vi "HTTPS Connection Callback.vi"(7 "Owner":refnum<class>, 8 "error in (no error)":errorcluster, 9 "Context":variant, 10 "Connection State":T1, 11 "Connection":refnum<class "Connection.lvclass">) -> (0 "error out":errorcluster)   [LabVIEW 2020, in "HTTP Server.lvlib" / "Server.lvclass"]
uses:
  Server.lvclass
  HTTP TCP Client/HTTP TCP Client.lvclass
  lv-stream/stream/Connection/Connection.lvclass
  lv-stream/stream/Connection State.ctl
  lv-stream/stream/Stream.lvlib
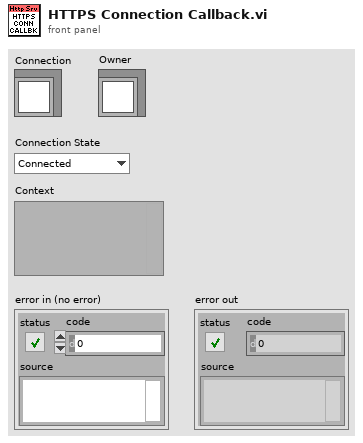
[diagram p1: front panel]
types:
  T1 = typedef "Stream.lvlib/Connection State.ctl" = enum16{"Connected", "Disconnected"}
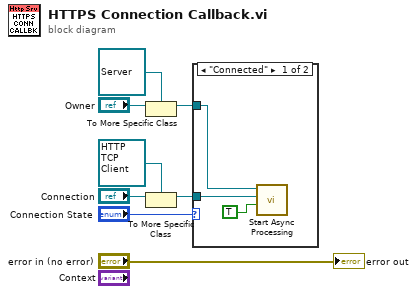
[diagram p0: block diagram]
diagram:
  n1 = To More Specific Class(target class=refnum<class "Server.lvclass"> refnum ("HTTP.lvlib:Server.lvclass"), reference="Owner") -> (specific class reference=w5:refnum<class "Server.lvclass">)  [unwired: 1 in, 1 out]
  n2 = To More Specific Class(target class=refnum<class "HTTP TCP Client.lvclass"> refnum ("HTTP Server.lvlib:HTTP TCP Client.lvclass"), reference="Connection") -> (specific class reference=w2:refnum<class "HTTP TCP Client.lvclass">)  [unwired: 1 in, 1 out]
  n3 = case shown="\"Connected\"" "Connection State" {
    tunnel: w5 -> [w11 _]
    tunnel: w2 -> [w10 _]
    frame "Connected" {
      n4 = call "Start Async Processing.vi"("HTTPS"=TRUE ("HTTPS?"), "Connection"=w10, "Server in"=w11) -> ()  [unwired: 7 in, 2 out]
    }
    frame "Disconnected" {
    }
  }
  "error out" <- "error in (no error)"
